vi "host.vi"() -> ()   [LabVIEW 2020]
uses:
  <vilib>/FPGAPlugInAG/cRIO-9035/niLvFpga_Open_cRIO-9035.vi
  <vilib>/rvi/interface/common/dynamic/niFpgaDynamicAddResources.vi
  <vilib>/Utility/error.llb/Error Cluster From Error Code.vi
  <vilib>/rvi/errors/niLvFpgaAdjustHostInterfaceError.vi
  <vilib>/FPGAPlugInAG/Dynamic/niLvFpga_Run_Dynamic.vi
  <vilib>/FPGAPlugInAG/Dynamic/niLvFpga_Close_Dynamic.vi
  <vilib>/rvi/interface/nirviOpenFPGA/nirviOpenFPGA.xnode
  FPGA Bitfiles/fftfpgaapplicati_FPGATarget_FFT2_jMgb+JE2xQs.lvbitx
  FFT.vi
  <vilib>/rvi/interface/nirviMethod/nirviMethod.xnode
  <vilib>/rvi/interface/nirviCloseFPGA/nirviCloseFPGA.xnode
  <vilib>/rvi/errors/niLvFpgaMergeErrorWithErrorCode.vi
  <vilib>/FPGAPlugInAG/Dynamic/niLvFpga_ReadFifo_Dynamic.vi
  <vilib>/FPGAPlugInAG/Dynamic/niLvFpga_WriteFifo_Dynamic.vi
  <vilib>/rvi/Analysis/host/Public/NI_FpgaMspHost.lvlib
panel:
  out "Array":fxp<+/-,32,16>[](array[numeric])
  out "magnitude 2":dbl[](array[numeric])
  out "size(s)":i32
  out "Magnitude":waveform(dbl)(graph)
  out "Spectrum":dbl[][](graph)
  out "df (Hz)":dbl
  out "end tick":fxp<+/-,32,16>[](array[numeric])
  out "start ticka":fxp<+/-,32,16>[](array[numeric])
  out "Waveform Graph":dbl[][](graph)
  out "input signal":T1(graph)
  out "MLP 1 size(s)":i32
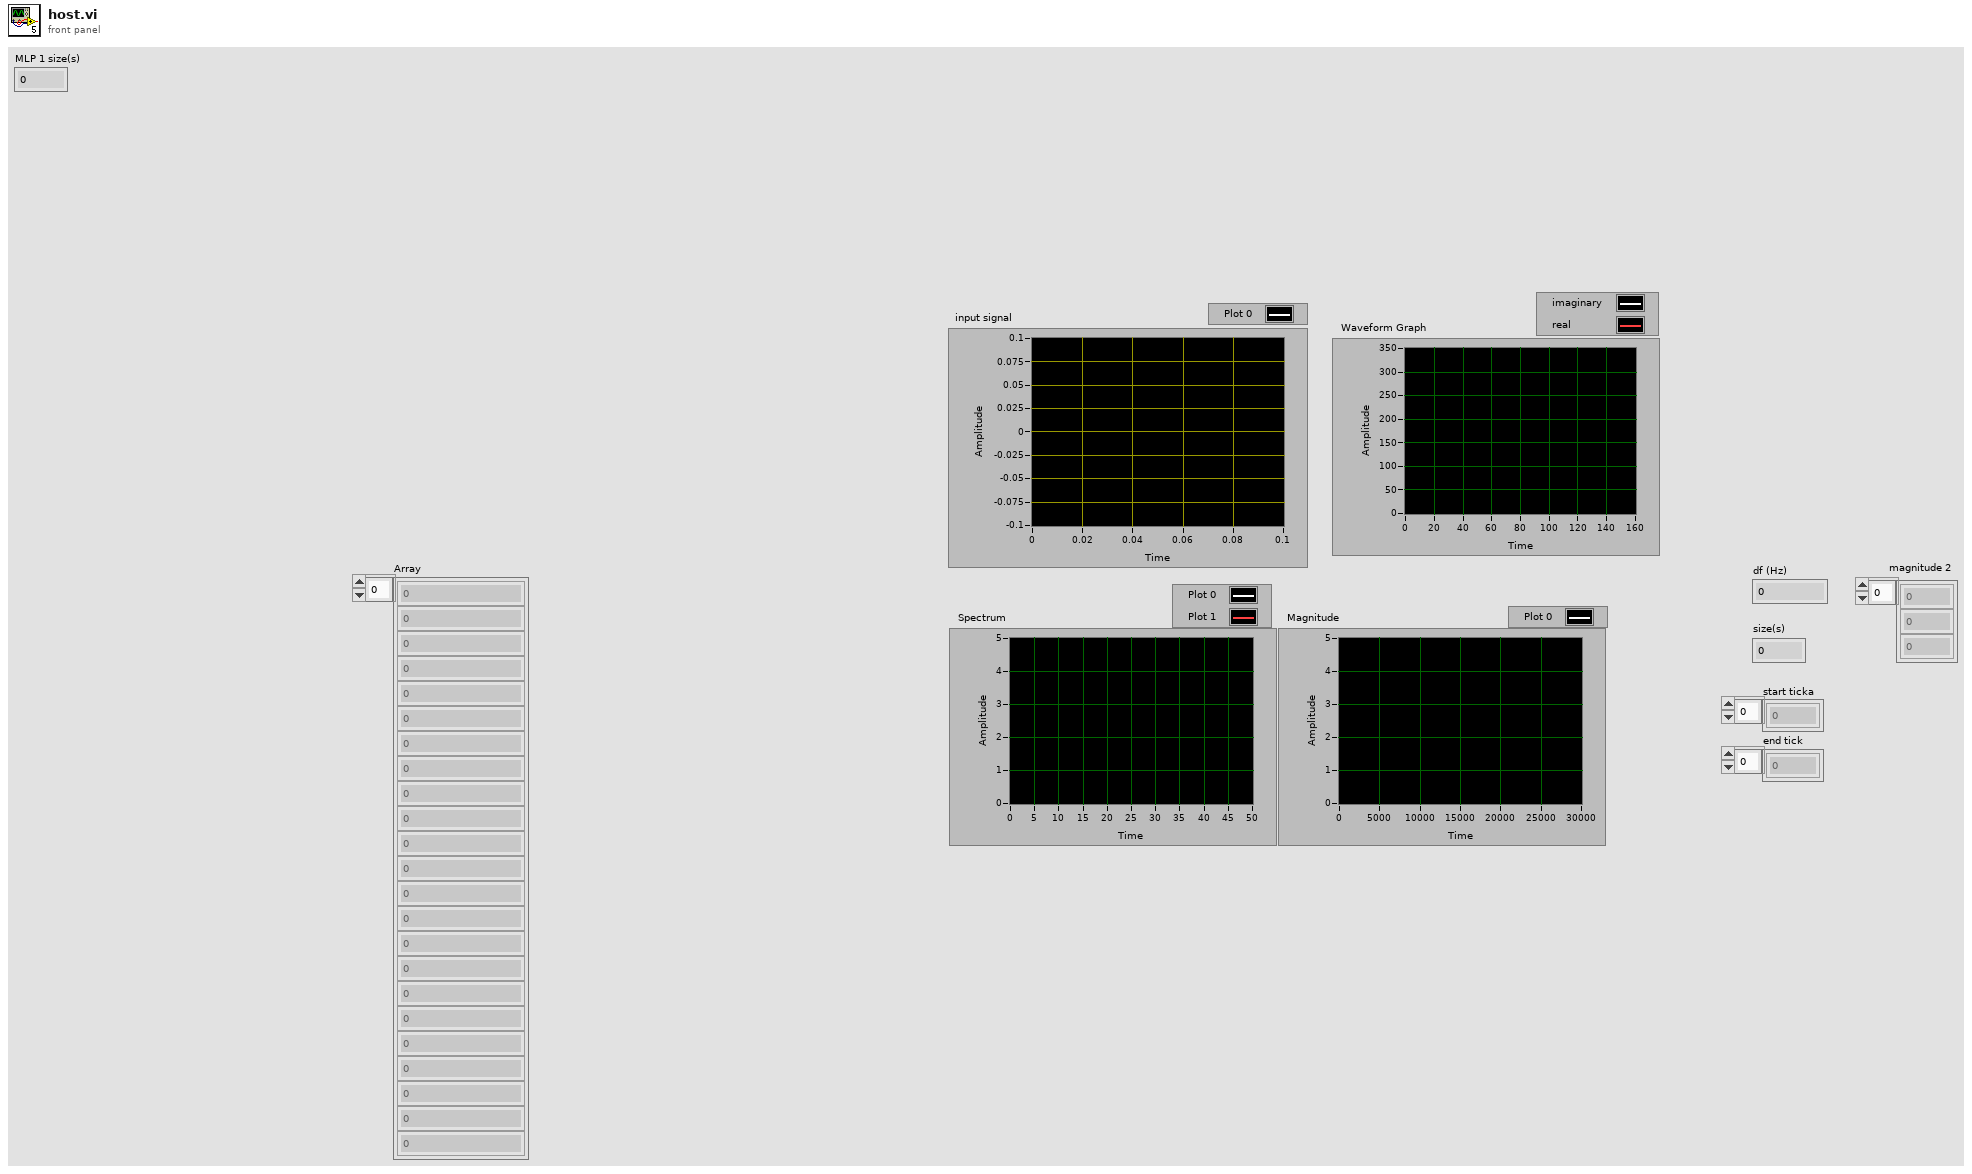
[diagram p1: front panel]
types:
  T1 = cluster{"array type (2D Dbl)":dbl[], "array type (2D Dbl)":dbl[]}
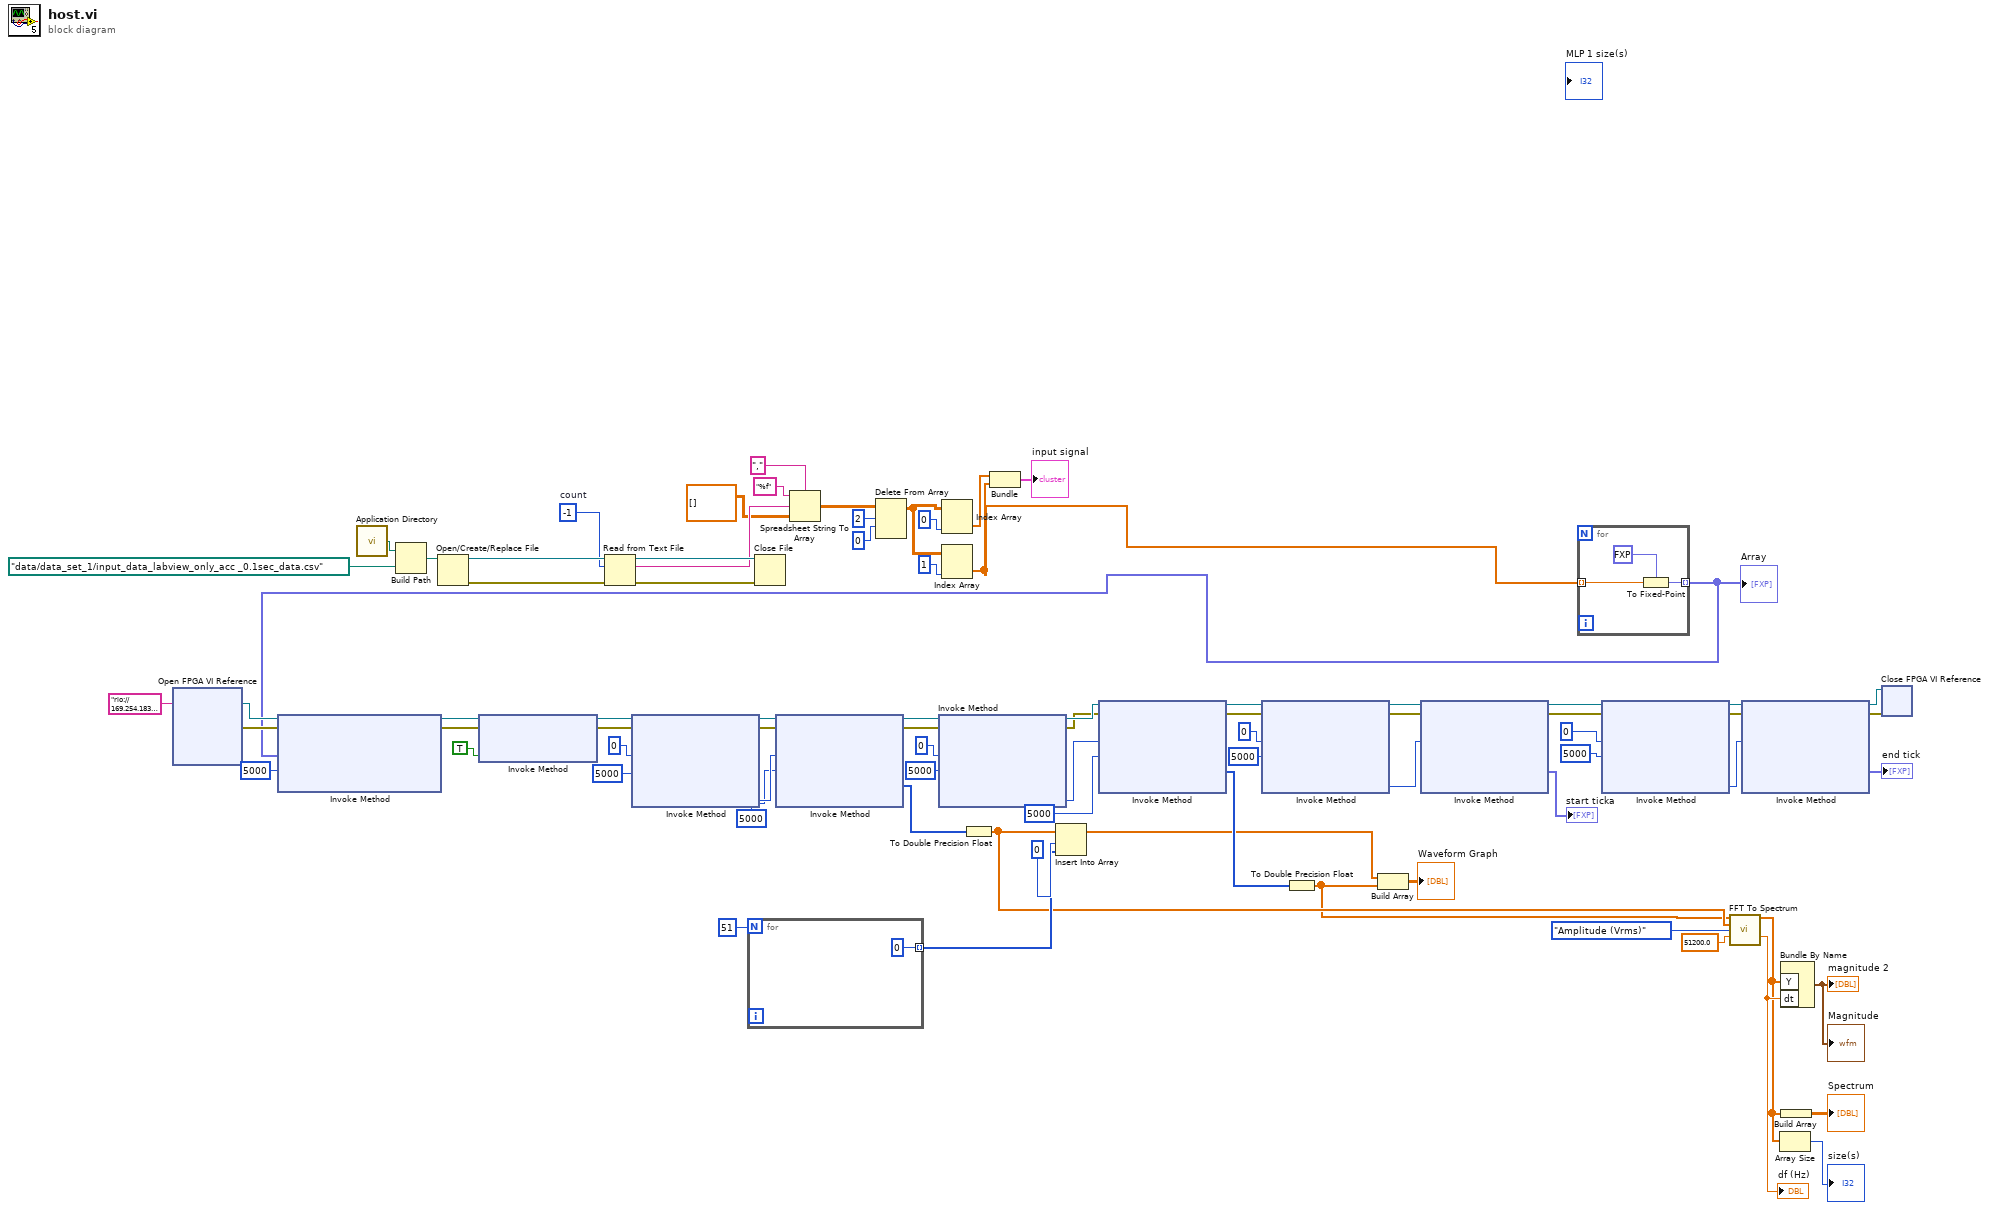
[diagram p0: block diagram]
diagram:
  w70 = -1  # count
  n1 = xnode "Open FPGA VI Reference"("resource name"=tag "rio://169.254.183.73/RIO0") -> ("FPGA VI Reference Out"=w60:refnum<k20>, "error out"=w59:errorcluster)  [unwired: 1 in]
  n2 = call <vilib>:"Application Directory.vi"() -> ("Application Directory"=w74:path)
  n3 = Build Path(base path=w74, name or relative path=path "data/data_set_1/input_data_labview_only_acc _0.1sec_data.csv" ("default name")) -> (appended path=w73:path)
  n4 = Open/Create/Replace File(file path (use dialog)=w73) -> (refnum out=w78:refnum<file>, error out=w79:errorcluster)  [unwired: 5 in, 1 out]
  n5 = Read from Text File(file (use dialog)=w78, count=w70, error in=w79) -> (refnum out=w77:refnum<file>, text=w75:string, error out=w76:errorcluster)  [unwired: 1 in, 1 out]
  n6 = for {
    N: 51 -> [_]
    tunnel: [0] -> w38 mode=indexing
  }
  n7 = Close File(refnum=w77, error in=w76) -> ()  [unwired: 2 out]
  n8 = Spreadsheet String To Array(delimiter (Tab)=",", format string="%f", spreadsheet string=w75, array type (2D Dbl)=dbl[][] []) -> (array=w67:dbl[][])
  n9 = Delete From Array(array=w67, length=2, index (row)=0) -> (array with subset deleted=w62:dbl[][])  [unwired: 1 in, 1 out]
  n10 = Index Array(array=w62, index (col)=0 ("disabled index (col)")) -> (element=w3:dbl[])  [unwired: 1 in]
  n11 = Index Array(array=w62, index (col)=1 ("disabled index (col)")) -> (element=w1:dbl[])  [unwired: 1 in]
  n12 = Bundle("array type (2D Dbl)"=w3, "array type (2D Dbl)"=w1) -> (→"input signal":T1)  [unwired: 1 in]
  n13 = for {
    tunnel: [w82] -> w2 mode=indexing
    tunnel: w1 -> [w81] mode=indexing
    n14 = To Fixed-Point(fixed-point type=fxp<+/-,32,16> 0.0 ("f"), number=w81) -> (fixed-point=w82:fxp<+/-,32,16>)
  }
  "Array" <- w2
  n15 = xnode "Invoke Method"("FPGA VI Reference In"=w60, "error in"=w59, "Data"=w2, "Timeout (ms)"=5000) -> ("FPGA VI Reference Out"=w57:refnum<k20>, "error out"=w56:errorcluster)  [unwired: 1 out]
  n16 = xnode "Invoke Method"("FPGA VI Reference In"=w57, "error in"=w56, "Wait Until Done (F)"=TRUE) -> ("FPGA VI Reference Out"=w55:refnum<k20>, "error out"=w54:errorcluster)
  n17 = xnode "Invoke Method"("FPGA VI Reference In"=w55, "error in"=w54, "Number of Elements"=u32 0, "Timeout (ms)"=5000) -> ("FPGA VI Reference Out"=w53:refnum<k20>, "error out"=w52:errorcluster, "Elements Remaining"=w46:u32)  [unwired: 1 out]
  n18 = xnode "Invoke Method"("FPGA VI Reference In"=w53, "error in"=w52, "Number of Elements"=w46, "Timeout (ms)"=5000) -> ("FPGA VI Reference Out"=w49:refnum<k20>, "error out"=w48:errorcluster, "Data"=w42:i32[])  [unwired: 1 out]
  n19 = xnode "Invoke Method"("FPGA VI Reference In"=w49, "error in"=w48, "Number of Elements"=u32 0, "Timeout (ms)"=5000) -> ("FPGA VI Reference Out"=w51:refnum<k20>, "error out"=w50:errorcluster, "Elements Remaining"=w44:u32)  [unwired: 1 out]
  n20 = To Double Precision Float(number=w42) -> (double precision float=w12:dbl[])
  n21 = Insert Into Array(array=w12, index=0, new element=w38) -> (w39:dbl[])
  n22 = xnode "Invoke Method"("FPGA VI Reference In"=w51, "error in"=w50, "Number of Elements"=w44, "Timeout (ms)"=5000) -> ("FPGA VI Reference Out"=w35:refnum<k20>, "error out"=w34:errorcluster, "Data"=w41:i32[])  [unwired: 1 out]
  n23 = xnode "Invoke Method"("FPGA VI Reference In"=w35, "error in"=w34, "Number of Elements"=u32 0, "Timeout (ms)"=5000) -> ("FPGA VI Reference Out"=w33:refnum<k20>, "error out"=w32:errorcluster, "Elements Remaining"=w25:u32)  [unwired: 1 out]
  n24 = To Double Precision Float(number=w41) -> (double precision float=w7:dbl[])
  n25 = Build Array(w39, w7) -> (→"Waveform Graph":dbl[][])
  n26 = xnode "Invoke Method"("FPGA VI Reference In"=w33, "error in"=w32, "Number of Elements"=w25) -> ("FPGA VI Reference Out"=w31:refnum<k20>, "error out"=w30:errorcluster, "Data"=→"start ticka":fxp<+/-,32,16>[])  [unwired: 1 in, 1 out]
  n27 = xnode "Invoke Method"("FPGA VI Reference In"=w31, "error in"=w30, "Number of Elements"=u32 0, "Timeout (ms)"=5000) -> ("FPGA VI Reference Out"=w29:refnum<k20>, "error out"=w28:errorcluster, "Elements Remaining"=w23:u32)  [unwired: 1 out]
  n28 = call <vilib>:"FFT To Spectrum.vi"("real FFT data"=w7, "imaginary FFT data"=w12, "spectrum type"=enum8{"Power (Vrms^2)", "Amplitude (Vrms)"}."Amplitude (Vrms)", "sample rate (S/s)"=51200.0) -> ("spectrum out"=w4:dbl[], "df (Hz)"=w6:dbl)  [unwired: 9 in, 1 out]
  "df (Hz)" <- w6
  n29 = xnode "Invoke Method"("FPGA VI Reference In"=w29, "error in"=w28, "Number of Elements"=w23) -> ("FPGA VI Reference Out"=w27:refnum<k20>, "error out"=w26:errorcluster, "Data"=→"end tick":fxp<+/-,32,16>[])  [unwired: 1 in, 1 out]
  n30 = Array Size(array=w4) -> (size(s)=→"size(s)":i32)
  n31 = Bundle By Name("Y"=w4, "dt"=w6) -> (→"Magnitude" →"magnitude 2":waveform(dbl))  [unwired: 1 in]
  n32 = Build Array(w4) -> (→"Spectrum":dbl[][])
  n33 = xnode "Close FPGA VI Reference"("FPGA VI Reference In"=w27, "error in"=w26) -> ()  [unwired: 1 out]
